vi "monedas counter.vi"(10 "numero de ciclos":i32, 11 "Array":dbl[](array[numeric])) -> (3 "Numeric":dbl)   [LabVIEW 2019]
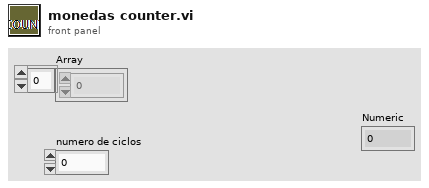
[diagram p1: front panel]
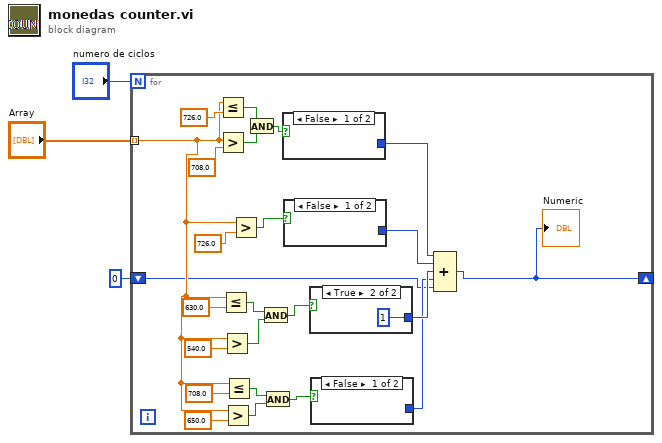
[diagram p0: block diagram]
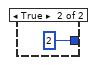
[diagram p2: hidden frame]
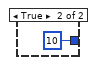
[diagram p4: hidden frame]
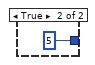
[diagram p5: hidden frame]
diagram:
  n1 = for {
    N: "numero de ciclos" -> [_]
    tunnel: "Array" -> [w15] mode=indexing
    shift-right: [w4] -> _
    shift-left: 0 -> [w5]
    n2 = Less Or Equal?(x=w15, y=726.0 ("x")) -> (x <= y?=w25:bool)
    n3 = Greater?(x=w15, y=708.0) -> (0:w26:bool)
    n4 = Less Or Equal?(x=w15, y=630.0) -> (x <= y?=w18:bool)
    n5 = Greater?(x=w15, y=540.0) -> (0:w17:bool)
    n6 = Greater?(x=w15, y=650.0) -> (0:w11:bool)
    n7 = Less Or Equal?(x=w15, y=708.0) -> (x <= y?=w12:bool)
    n8 = Greater?(x=w15, y=726.0) -> (0:w21:bool)
    n9 = And(x=w25, y=w26) -> (x .and. y?=w24:bool)
    n10 = And(x=w18, y=w17) -> (x .and. y?=w16:bool)
    n11 = And(x=w12, y=w11) -> (x .and. y?=w10:bool)
    n12 = case shown="False" w24 {
      tunnel: [_ 5] -> w9
      frame False {
      }
      frame True {
      }
    }
    n13 = case shown="False" w21 {
      tunnel: [_ 10] -> w8
      frame False {
      }
      frame True {
      }
    }
    n14 = case shown="True" w16 {
      tunnel: [_ 1] -> w7
      frame False {
      }
      frame True {
      }
    }
    n15 = case shown="False" w10 {
      tunnel: [_ 2] -> w6
      frame False {
      }
      frame True {
      }
    }
    n16 = Compound Arithmetic op=ADD(w9, w8, w7, w6, w5) -> (w4:i32)
    "Numeric" <- w4
  }
